vi "AIT 664 Tx Message Ports Page.vi"(8 "error in (no error)":errorcluster, 11 "Node Ptr":T2 format="%.0x") -> (0 "error out":errorcluster)   [LabVIEW 2013, in "AIT 664 Custom Device.lvlib"]
uses:
  AIT 664 Custom Device.lvlib
  <vilib>/NI Veristand/Custom Device API/Custom Device Item Ref.ctl
  Controls/664 - Sampling Type.ctl
  Controls and Global/Global.vi
  <vilib>/NI Veristand/Custom Device API/Get Item Property (U32).vi
  <vilib>/NI Veristand/Custom Device API/Get Item Property (String).vi
  <vilib>/NI Veristand/Custom Device API/Get Item Property (Variant).vi
  <vilib>/NI Veristand/Custom Device API/Set Item Property (U32).vi
  <vilib>/NI Veristand/Custom Device API/Custom Device API.lvlib
panel:
  in  "Tx Rate (ms)":u32
  out "Destination UDP Port":u32
  out "Destination IP Address":string
  out "Source UDP Port":u32
  out "Source IP Address":string
  out "Sampling Type":T1
  out "Port Id":u32
  in  "Header":cluster{"Section Name":string}={"Section Name"="AIT 664 Tx Message Ports Page"}
  in  "Description":string
  out "Name":string
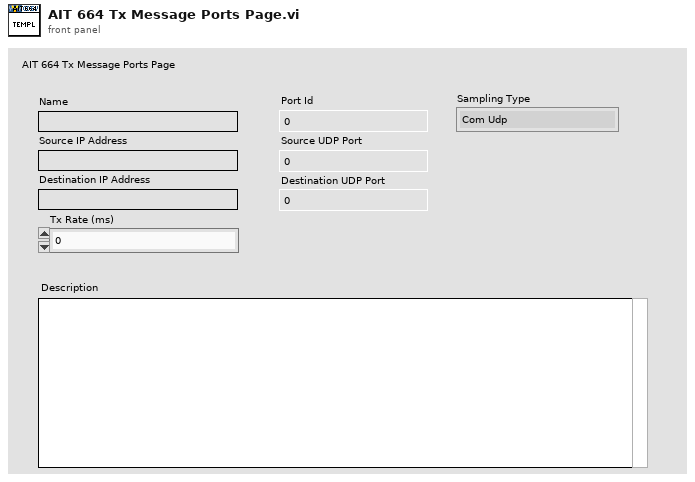
[diagram p1: front panel]
types:
  T1 = typedef "AIT 664 Custom Device.lvlib/664 - Sampling Type.ctl" = enum16{"Com Udp", "Com Udp Queuing", "Sap Udp", "Sap Ip", "Sap Mac", "Unknown"}
  T2 = typedef "Custom Device API.lvlib/Custom Device Item Ref.ctl" = u64
  T3 = typedef "Custom Device API.lvlib/Custom Device Item Info.ctl" = cluster{"Name":string, "Is Channel":bool, "GUID":string, "Is Waveform":bool}
  T4 = typedef "Custom Device API.lvlib/Custom Device Commands.ctl" = enum16{"Default", "Item renamed", "Shutdown", "Dynamic button pressed"}
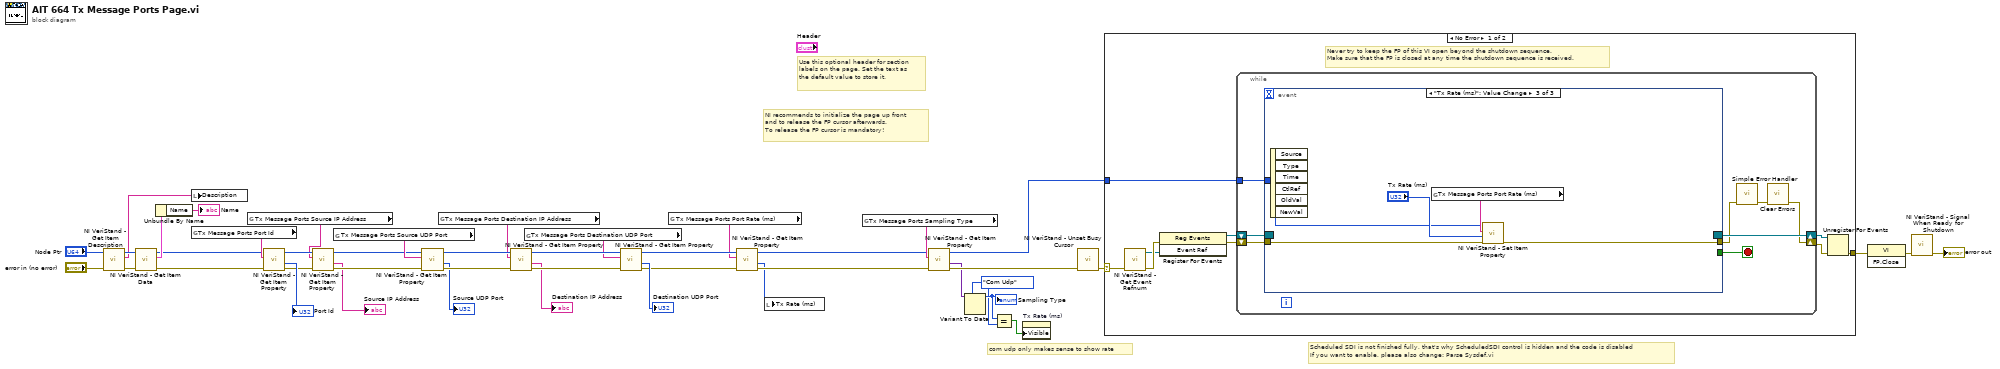
[diagram p0: block diagram]
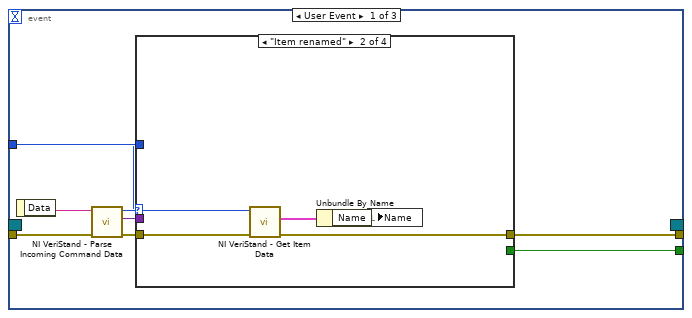
[diagram p2: hidden frame]
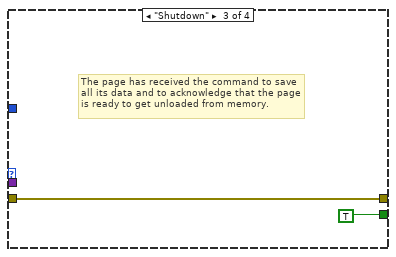
[diagram p4: hidden frame]
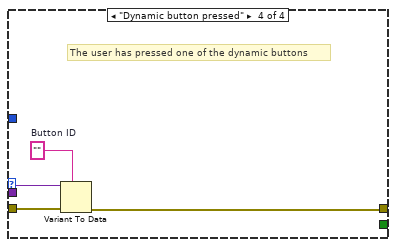
[diagram p5: hidden frame]
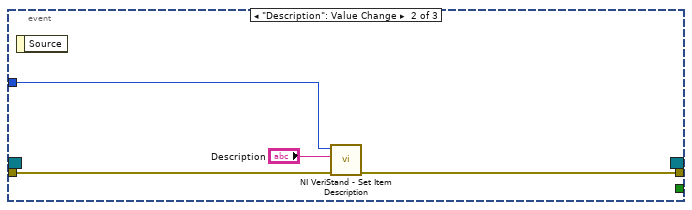
[diagram p6: hidden frame]
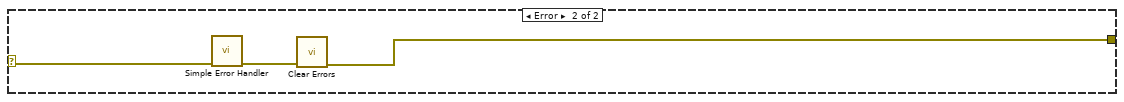
[diagram p7: hidden frame]
diagram:
  w2 = 664_-_Sampling_Type."Com Udp" ("Sampling Type")
  # "com udp only makes sense to show rate"
  # "Scheduled SDI is not finished fully, that's why ScheduledSDI control is hidden and the code is disabled\nIf you want to enable, please also change: Parse Sysdef.vi"
  # "Use this optional header for section labels on the page. Set the text as the default value to store it."
  # "NI recommends to initialize the page up front\nand to release the FP cursor afterwards.\nTo release the FP cursor is mandatory!"
  n1 = call <vilib>:"NI VeriStand - Get Item Description.vi"("error in (no error)"="error in (no error)", "Item Ref in"="Node Ptr") -> ("error out"=w38:errorcluster, "Description"=w39:string, "Item Ref out"=w40:T2)  [unwired: 7 out]
  n2 = call <vilib>:"NI VeriStand - Get Item Data.vi"("error in (no error)"=w38, "Item Ref in"=w40) -> ("error out"=w31:errorcluster, "Item Info"=w37:T3, "Item Ref out"=w30:T2)  [unwired: 7 out]
  n3 = Unbundle By Name(w37) -> ("Name"=→"Name":string)
  n4 = local write "Description"(w39) -> ()
  n5 = global read "Global.vi" "Tx Message Ports Port Id"() -> (w32:string)
  n6 = global read "Global.vi" "Tx Message Ports Source IP Address"() -> (w14:string)
  n7 = call-poly <vilib>:"NI VeriStand - Get Item Property.vi"("error in (no error)"=w31, "Property Name"=w32, "Item Ref in"=w30) -> ("error out"=w16:errorcluster, "Value"=→"Port Id":u32, "Item Ref out"=w15:T2)  [unwired: 5 in, 1 out]
  n8 = call-poly <vilib>:"NI VeriStand - Get Item Property.vi"("error in (no error)"=w16, "Property Name"=w14, "Item Ref in"=w15) -> ("error out"=w17:errorcluster, "Value"=→"Source IP Address":string, "Item Ref out"=w18:T2)  [unwired: 5 in, 1 out]
  n9 = global read "Global.vi" "Tx Message Ports Source UDP Port"() -> (w19:string)
  n10 = call-poly <vilib>:"NI VeriStand - Get Item Property.vi"("error in (no error)"=w17, "Property Name"=w19, "Item Ref in"=w18) -> ("error out"=w24:errorcluster, "Value"=→"Source UDP Port":u32, "Item Ref out"=w25:T2)  [unwired: 5 in, 1 out]
  n11 = global read "Global.vi" "Tx Message Ports Destination IP Address"() -> (w23:string)
  n12 = call-poly <vilib>:"NI VeriStand - Get Item Property.vi"("error in (no error)"=w24, "Property Name"=w23, "Item Ref in"=w25) -> ("error out"=w22:errorcluster, "Value"=→"Destination IP Address":string, "Item Ref out"=w21:T2)  [unwired: 5 in, 1 out]
  n13 = global read "Global.vi" "Tx Message Ports Destination UDP Port"() -> (w20:string)
  n14 = call-poly <vilib>:"NI VeriStand - Get Item Property.vi"("error in (no error)"=w22, "Property Name"=w20, "Item Ref in"=w21) -> ("error out"=w9:errorcluster, "Value"=→"Destination UDP Port":u32, "Item Ref out"=w7:T2)  [unwired: 5 in, 1 out]
  n15 = global read "Global.vi" "Tx Message Ports Port Rate (ms)"() -> (w5:string)
  n16 = call-poly <vilib>:"NI VeriStand - Get Item Property.vi"("error in (no error)"=w9, "Property Name"=w5, "Item Ref in"=w7) -> ("error out"=w8:errorcluster, "Value"=w4:u32, "Item Ref out"=w6:T2)  [unwired: 5 in, 1 out]
  n17 = local write "Tx Rate (ms)"(w4) -> ()
  n18 = global read "Global.vi" "Tx Message Ports Sampling Type"() -> (w27:string)
  n19 = call-poly <vilib>:"NI VeriStand - Get Item Property.vi"("error in (no error)"=w8, "Property Name"=w27, "Item Ref in"=w6) -> ("error out"=w29:errorcluster, "Value"=w26:variant, "Item Ref out"=w28:T2)  [unwired: 5 in, 1 out]
  n20 = Variant To Data(type=w2, Variant=w26) -> (data=w3:T1)  [unwired: 1 in, 1 out]
  "Sampling Type" <- w3
  n21 = Equal?(x=w3, y=w2) -> (x = y?=w1:bool)
  n22 = property on="Tx Rate (ms)" class="DigNum (strict)"("Visible"=w1) -> ()  [unwired: 2 in, 2 out]
  n23 = call <vilib>:"NI VeriStand - Unset Busy Cursor.vi"("error in (no error)"=w29) -> ("error out"=w41:errorcluster)  [unwired: 10 out]
  n24 = case shown="No Error" w41 {
    selector: w41 -> [w45 w93]
    tunnel: [w50 w91] -> w44
    tunnel: w28 -> [w46 _]
    frame No Error {
      # "Never try to keep the FP of this VI open beyond the shutdown sequence.\nMake sure that the FP is closed at any time the shutdown sequence is received."
      n25 = call <vilib>:"NI VeriStand - Get Event Refnum.vi"("error in (no error)"=w45) -> ("error out"=w53:errorcluster, "Event Ref"=w49:refnum<user-event>)  [unwired: 9 out]
      n26 = register-events(error in=w53, w49) -> (reference out=w47:refnum<event-registration>, error out=w48:errorcluster)  [unwired: 1 in]
      n27 = while {
        tunnel: w46 -> [w57]
        shift-right: [w54] -> w51
        shift-left: w48 -> [w60]
        shift-right: [w61] -> w52
        shift-left: w47 -> [w59]
        stop <- w58 stop-if-true
        n28 = event shown="[2] \"Tx Rate (ms)\": Value Change" {
          selector: w59 -> [_ _ _]
          dyn-events: [_ _ _] -> w61
          timeout: _ -> [_ _ _]
          tunnel: w60 -> [w69 w84 w90]
          tunnel: [w65 _ _] -> w58
          tunnel: [w64 w83 w89] -> w56
          tunnel: w57 -> [w63 w85 w86]
          event User Event {
            n29 = event-data() -> ("Data"=w68:string)  [unwired: 1 out]
            n30 = call <vilib>:"NI VeriStand - Parse Incoming Command Data.vi"("error in (no error)"=w69, "Incoming data"=w68) -> ("error out"=w67:errorcluster, "Outgoing data"=w62:variant, "Action"=w66:T4)  [unwired: 7 out]
            n31 = case shown="\"Item renamed\"" w66 {
              tunnel: w67 -> [w70 w75 w76 w81]
              tunnel: [_ _ TRUE _] -> w65
              tunnel: [w70 w72 w76 w78] -> w64
              tunnel: w63 -> [_ w74 _ _]
              tunnel: w62 -> [_ _ _ w80]
              frame "Default", Default {
              }
              frame "Item renamed" {
                n32 = call <vilib>:"NI VeriStand - Get Item Data.vi"("error in (no error)"=w75, "Item Ref in"=w74) -> ("error out"=w72:errorcluster, "Item Info"=w73:T3)  [unwired: 8 out]
                n33 = Unbundle By Name(w73) -> ("Name"=w71:string)
                n34 = local write "Name"(w71) -> ()
              }
              frame "Shutdown" {
                # "The page has received the command to save all its data and to acknowledge that the page is ready to get unloaded from memory."
              }
              frame "Dynamic button pressed" {
                w79 = ""  # Button ID
                # "The user has pressed one of the dynamic buttons"
                n35 = Variant To Data(error in=w81, type=w79, Variant=w80) -> (error out=w78:errorcluster)  [unwired: 1 out]
              }
            }
          }
          event "Description": Value Change {
            n36 = event-data() -> ()  [unwired: 2 out]
            n37 = call <vilib>:"NI VeriStand - Set Item Description.vi"("error in (no error)"=w84, "Description"="Description", "Item Ref in"=w85) -> ("error out"=w83:errorcluster)  [unwired: 8 out]
          }
          event "Tx Rate (ms)": Value Change {
            n38 = event-data() -> ()  [unwired: 7 out]
            n39 = global read "Global.vi" "Tx Message Ports Port Rate (ms)"() -> (w88:string)
            n40 = call-poly <vilib>:"NI VeriStand - Set Item Property.vi"("error in (no error)"=w90, "Value"="Tx Rate (ms)", "Property Name"=w88, "Item Ref in"=w86) -> ("error out"=w89:errorcluster)  [unwired: 5 in, 2 out]
          }
        }
        n41 = call <vilib>:"Simple Error Handler.vi"("error in (no error)"=w56) -> ("error out"=w55:errorcluster)  [unwired: 1 in, 7 out]
        n42 = call <vilib>:"Clear Errors.vi"("error in (no error)"=w55) -> ("error out"=w54:errorcluster)  [unwired: 6 out]
      }
      n43 = Unregister For Events(event registration refnum=w52, error in=w51) -> (error out=w50:errorcluster)
    }
    frame Error {
      n44 = call <vilib>:"Simple Error Handler.vi"("error in (no error)"=w93) -> ("error out"=w92:errorcluster)  [unwired: 1 in, 7 out]
      n45 = call <vilib>:"Clear Errors.vi"("error in (no error)"=w92) -> ("error out"=w91:errorcluster)  [unwired: 6 out]
    }
  }
  n46 = invoke class="VI" method="FP.Close"(error in=w44) -> (error out=w43:errorcluster)  [unwired: 2 in, 2 out]
  n47 = call <vilib>:"NI VeriStand - Signal When Ready for Shutdown.vi"("error in (no error)"=w43) -> ("error out"=→"error out":errorcluster)  [unwired: 10 out]
